vi "[SubVI]Locmotion_Mode.vi"(6 "Mode Input":enum32{"LG", "RA", "RD", "SA", "SD"}(ring), 7 "RA Assist Mode":enum16{"Static", "Scaled"}(ring), 8 "Ramp Incline Level":enum16{"Ramp 4", "Ramp 3", "Ramp 2", "Ramp 1"}(ring), 9 "Assist Percent":dbl, 10 "Body Weight":dbl) -> (1 "Ext Set":dbl, 2 "Flex Set":dbl, 3 "Walking Mode":i32)   [LabVIEW 2019]
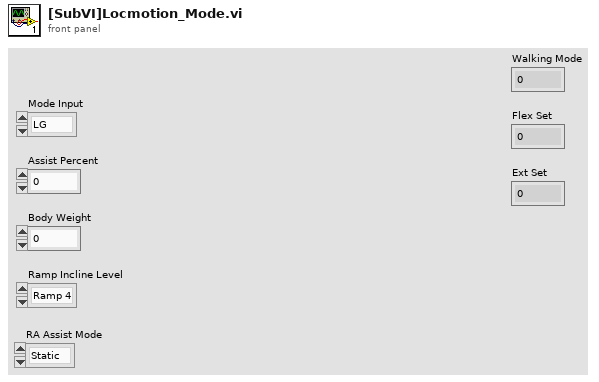
[diagram p1: front panel]
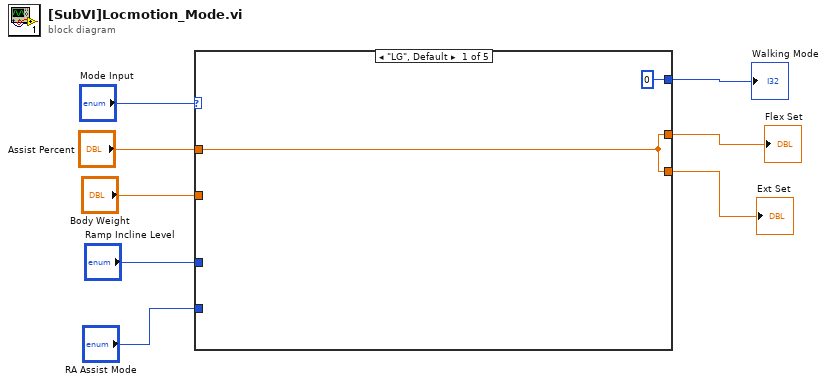
[diagram p0: block diagram]
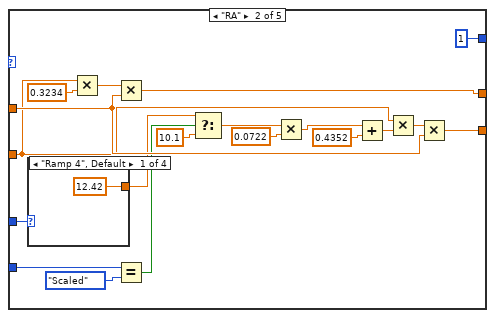
[diagram p2: hidden frame]
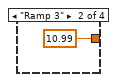
[diagram p3: hidden frame]
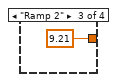
[diagram p4: hidden frame]
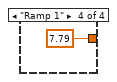
[diagram p5: hidden frame]
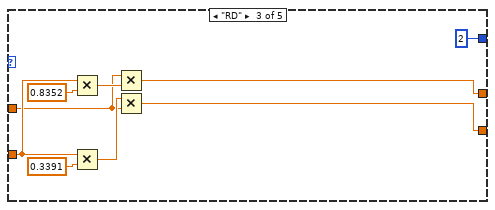
[diagram p6: hidden frame]
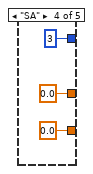
[diagram p7: hidden frame]
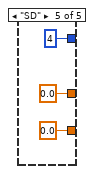
[diagram p8: hidden frame]
diagram:
  n1 = case shown="\"LG\", Default" "Mode Input" {
    tunnel: [0 1 2 3 4] -> w2
    tunnel: "Ramp Incline Level" -> [_ w28 _ _ _]
    tunnel: [w9 w18 w34 0.0 ("y") 0.0 ("y")] -> w4
    tunnel: [w9 w17 w37 0.0 ("y") 0.0 ("y")] -> w5
    tunnel: "Assist Percent" -> [w9 w20 w35 _ _]
    tunnel: "Body Weight" -> [_ w19 w39 _ _]
    tunnel: "RA Assist Mode" -> [_ w16 _ _ _]
    frame "LG", Default {
    }
    frame "RA" {
      n2 = case shown="\"Ramp 4\", Default" w28 {
        tunnel: [12.42 ("Flexion Torque 2") 10.99 ("Flexion Torque 2") 9.21 ("Flexion Torque 2") 7.79 ("Flexion Torque 2")] -> w12
        frame "Ramp 4", Default {
        }
        frame "Ramp 3" {
        }
        frame "Ramp 2" {
        }
        frame "Ramp 1" {
        }
      }
      n3 = Multiply(x=w19, y=0.3234) -> (x*y=w27:dbl)
      n4 = Multiply(x=w27, y=w20) -> (x*y=w17:dbl)
      n5 = Equal?(x=w16, y=enum16{"Static", "Scaled"}."Scaled") -> (x = y?=w14:bool)
      n6 = Select(t=w12, s=w14, f=10.1) -> (s? t:f=w13:dbl)
      n7 = Multiply(x=w13, y=0.0722 ("Flexion Torque 2")) -> (x*y=w22:dbl)
      n8 = Add(x=w22, y=0.4352) -> (x+y=w25:dbl)
      n9 = Multiply(x=w19, y=w25) -> (x*y=w24:dbl)
      n10 = Multiply(x=w24, y=w20) -> (x*y=w18:dbl)
    }
    frame "RD" {
      n11 = Multiply(x=w39, y=0.8352) -> (x*y=w38:dbl)
      n12 = Multiply(x=w39, y=0.3391) -> (x*y=w36:dbl)
      n13 = Multiply(x=w35, y=w38) -> (x*y=w37:dbl)
      n14 = Multiply(x=w36, y=w35) -> (x*y=w34:dbl)
    }
    frame "SA" {
    }
    frame "SD" {
    }
  }
  "Flex Set" <- w5
  "Ext Set" <- w4
  "Walking Mode" <- w2
